vi "LogLookUpScale.vi"(10 "Log Lookup":sgl[](array[numeric]), 11 "Array in":dbl[][](array[numeric])) -> (3 "Array out":sgl[][](array[numeric]))   [LabVIEW 2022 SP3]
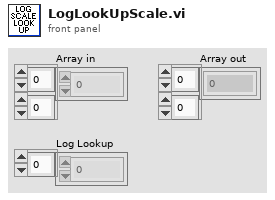
[diagram p1: front panel]
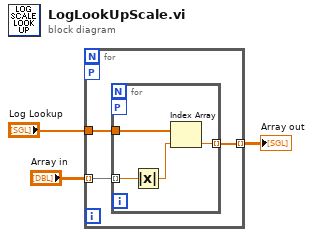
[diagram p0: block diagram]
diagram:
  n1 = for {
    tunnel: [w6] -> w1 mode=indexing
    tunnel: "Array in" -> [w5] mode=indexing
    workers-P: _ -> [_]
    tunnel: "Log Lookup" -> [w4]
    n2 = for {
      tunnel: [w10] -> w6 mode=indexing
      tunnel: w5 -> [w9] mode=indexing
      workers-P: _ -> [_]
      tunnel: w4 -> [w7]
      n3 = Absolute Value(x=w9) -> (abs(x)=w8:dbl)
      n4 = Index Array(array=w7, index=w8) -> (element=w10:sgl)
    }
  }
  "Array out" <- w1
